vi "initialize_SPIMCams_Param_Adjust_(SubVI).vi"(8 "Image Name":string="stream", 9 "Cam A ROI":T4, 10 "Cam B ROI":T4, 11 "Camera select":u16) -> (0 "error out":errorcluster, 1 "Buffer Info":T2, 2 "IMAQ error out":errorcluster, 3 "IMAQ image out":T1, 4 "Handle out":u32, 5 "Camera Details":T3)   [LabVIEW 2016]
uses:
  <vilib>/vision/Image Controls.llb/IMAQ Image.ctl
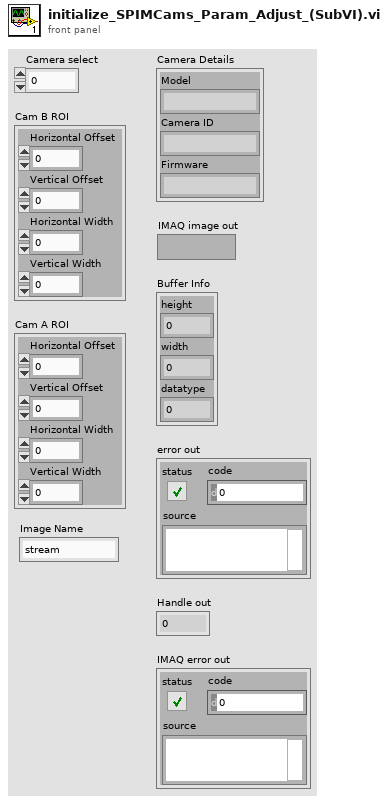
[diagram p1: front panel]
types:
  T1 = typedef "IMAQ Image.ctl" = refnum<image>
  T2 = cluster{"height":u32, "width":u32, "datatype":u32}
  T3 = cluster{"Model":string, "Camera ID":string, "Firmware":string}
  T4 = cluster{"Horizontal Offset":i32, "Vertical Offset":i32, "Horizontal Width":i32, "Vertical Width":i32}
  T5 = cluster{"height":i32, "width":i32, "datatype":i32}
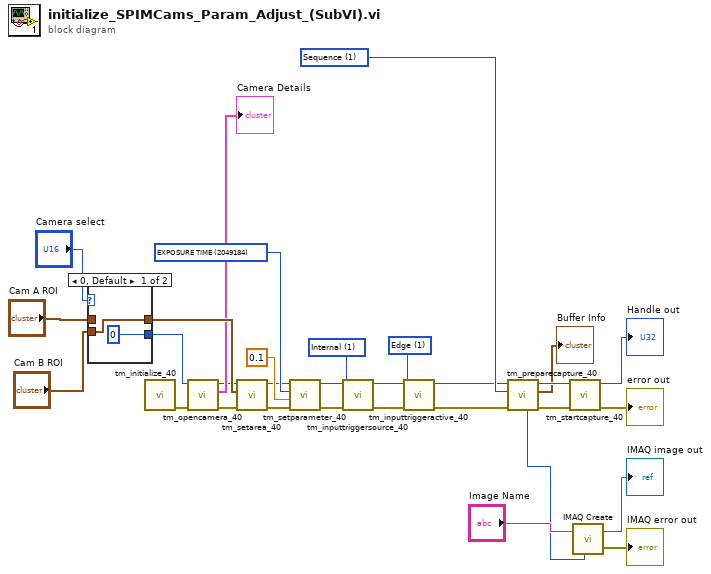
[diagram p0: block diagram]
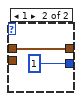
[diagram p2: hidden frame]
diagram:
  w3 = 1 items=["Edge"=1, "Level"=2, "Sync Readout"=3, "Point"=4] ("Active")
  w4 = 1 items=["Internal"=1, "External"=2, "Software"=3, "Master Pulse"=4] ("Source")
  w18 = u32 2049184 items=["SENSOR MODE"=4212128, "CCD MODE"=4212384, "READOUT MODE"=4211872, "ACTIVE VIEW INDEX"=4343136, "BITS PER CHANNEL"=4342976, "IMAGE PIXEL TYPE"=4343296, "BINNING"=4215968, "EXPOSURE TIME"=2049184, "CONTRAST GAIN"=3163312, "CONTRAST OFFSET"=3163328, "LIGHT MODE"=2114720, "SENSITIVITY"=2114992, "PHOTON IMAGING MODE"=2115200, "HIGH DYNAMIC RANGE MODE"=3163360, "WHITE BALANCE"=3163568, "TEMPERATURE"=2115232, "TEMPERATURE TARGET"=2115264, "SENSOR COOLER FAN"=2115296, "LINEBUNDLE HEIGHT"=4212192, "MECHANICAL SHUTTER"=2115488, "BACK FOCUS POSITION"=8422304, "TRIGGER CONNECTOR"=1066432, "TRIGGER SOURCE"=1066144, "OUTPUT TRIGGER SOURCE"=1852576, "TRIGGER GLOBAL EXPOSURE"=2049680, "FIRST TRIGGER BEHAVIOR"=2049696, "CHANNEL SYNC"=1852352, "READOUT DIRECTION"=4211904, "PRE HSYNC COUNT"=1852704, "INTERNAL LINE SPEED"=4226000, "INTERNAL LINE INTERVAL"=4226016] ("Parameter")
  w21 = 1 items=["Snap", "Sequence"] ("Capture mode")
  n1 = case shown="0, Default" "Camera select" {
    tunnel: [0 1] -> w28
    tunnel: "Cam A ROI" -> [_ w34]
    tunnel: [w32 w34] -> w27
    tunnel: "Cam B ROI" -> [w32 _]
    frame 0, Default {
    }
    frame 1 {
    }
  }
  n2 = call <userlib>:"tm_initialize_40.vi"() -> ("error out"=w26:errorcluster)  [unwired: 8 in, 3 out]
  n3 = call <userlib>:"tm_opencamera_40.vi"("error in (no error)"=w26, "Camera Index"=w28) -> ("error out"=w24:errorcluster, "Camera Details"=→"Camera Details":T3, "Handle out"=w23:u32)  [unwired: 7 in]
  n4 = call <userlib>:"tm_setarea_40.vi"("error in (no error)"=w24, "Sub Region"=w27, "Handle in"=w23) -> ("error out"=w9:errorcluster, "Handle out"=w10:u32)  [unwired: 7 in]
  n5 = call <userlib>:"tm_setparameter_40.vi"("error in (no error)"=w9, "Value in"=0.1, "Parameter"=w18, "Handle in"=w10) -> ("error out"=w8:errorcluster, "Handle out"=w7:u32)  [unwired: 6 in]
  n6 = call <userlib>:"tm_inputtriggersource_40.vi"("error in (no error)"=w8, "Source"=w4, "Handle in"=w7) -> ("error out"=w6:errorcluster, "Handle out"=w5:u32)  [unwired: 7 in]
  n7 = call <userlib>:"tm_inputtriggeractive_40.vi"("error in (no error)"=w6, "Active"=w3, "Handle in"=w5) -> ("error out"=w1:errorcluster, "Handle out"=w2:u32)  [unwired: 7 in]
  n8 = call <userlib>:"tm_preparecapture_40.vi"("error in (no error)"=w1, "Capture mode"=w21, "Handle in"=w2) -> ("error out"=w19:errorcluster, "Buffer Info"=→"Buffer Info":T5, "Handle out"=w20:u32, "Image type"=w11:u32)  [unwired: 5 in]
  n9 = call <userlib>:"tm_startcapture_40.vi"("error in (no error)"=w19, "Handle in"=w20) -> ("error out"=→"error out":errorcluster, "Handle out"=→"Handle out":u32)  [unwired: 8 in]
  n10 = call "IMAQ Create"("Image Name"="Image Name", "Image Type"=w11) -> ("New Image"=→"IMAQ image out":T1, "error out"=→"IMAQ error out":errorcluster)  [unwired: 3 in]
